vi "svl_Low Pass [Order 1] No State.vi"(6 "state info in":T1 {"y(n-2) state" format="%.2f"; "x(n-2) state" format="%.2f"; "y(n-1) state" format="%.2f"; "x(n-1) state" format="%.2f"}, 9 "reset":bool=TRUE, 10 "filter coefficients":cluster{"beta":dbl, "gamma":dbl, "alpha":dbl} {"alpha" format="%.2f"; "gamma" format="%.2f"; "beta" format="%.2f"}, 11 "Input stream":dbl[](array[numeric])) -> (3 "filtered signal":dbl[](array[numeric]), 4 "state info out":T1 {"y(n-2) state" format="%.2f"; "x(n-2) state" format="%.2f"; "y(n-1) state" format="%.2f"; "x(n-1) state" format="%.2f"})   [LabVIEW 2017, in "SoundVib_Integration.lvlib"]
uses:
  <vilib>/addons/Sound and Vibration/svt_Integration/SoundVib_Integration.lvlib
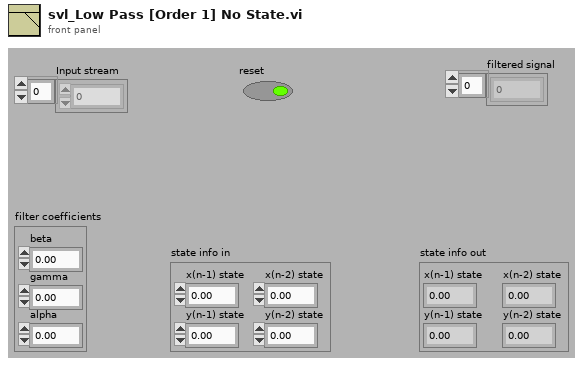
[diagram p1: front panel]
types:
  T1 = cluster{"x(n-1) state":dbl, "y(n-1) state":dbl, "x(n-2) state":dbl, "y(n-2) state":dbl}
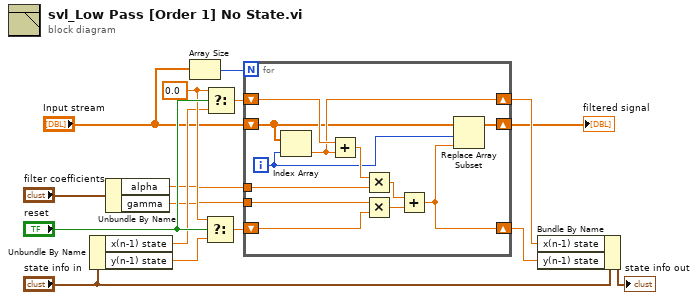
[diagram p0: block diagram]
diagram:
  w10 = 0.0 ("Element Data")
  n1 = Unbundle By Name("state info in") -> ("x(n-1) state"=w8:dbl, "y(n-1) state"=w12:dbl)
  n2 = Unbundle By Name("filter coefficients") -> ("alpha"=w6:dbl, "gamma"=w5:dbl)
  n3 = Array Size(array="Input stream") -> (size(s)=w4:i32)
  n4 = Select(t=w10, s="reset", f=w12) -> (s? t:f=w9:dbl)
  n5 = Select(t=w10, s="reset", f=w8) -> (s? t:f=w11:dbl)
  n6 = for {
    N: w4 -> [_]
    shift-right: [w21] -> w13
    shift-left: w11 -> [w28]
    tunnel: w6 -> [w22]
    shift-right: [w18] -> w14
    shift-left: w9 -> [w24]
    tunnel: w5 -> [w26]
    shift-right: [w19] -> w1
    shift-left: "Input stream" -> [w20]
    i -> [w17]
    n7 = Index Array(array=w20, index=w17) -> (element=w21:dbl)
    n8 = Add(x=w28, y=w21) -> (x+y=w27:dbl)
    n9 = Multiply(x=w27, y=w22) -> (x*y=w23:dbl)
    n10 = Multiply(x=w26, y=w24) -> (x*y=w25:dbl)
    n11 = Add(x=w23, y=w25) -> (x+y=w18:dbl)
    n12 = Replace Array Subset(array=w20, new element=w18, index=w17) -> (w19:dbl[])
  }
  "filtered signal" <- w1
  n13 = Bundle By Name(cluster="state info in", "x(n-1) state"=w13, "y(n-1) state"=w14) -> (→"state info out":T1)
